vi "WaitOnCommand.vi"(7 "timeout in ms (-1)":i32, 8 "error in (no error)":errorcluster, 10 "queue out":refnum<queue>, 11 "Subsystem in":refnum<class "Subsystem.lvclass">) -> (0 "error out":errorcluster, 2 "element":refnum<class "SubsystemData.lvclass">, 3 "Subsystem out":refnum<class "Subsystem.lvclass">)   [LabVIEW 2017, in "Subsystem.lvclass"]
uses:
  Subsystem.lvclass
  SubsystemData/SubsystemData.lvclass
  Subsystem.lvclass/Subsystem.ctl
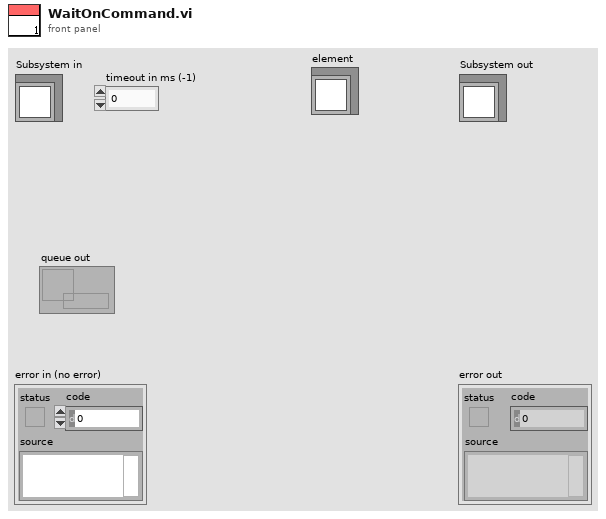
[diagram p1: front panel]
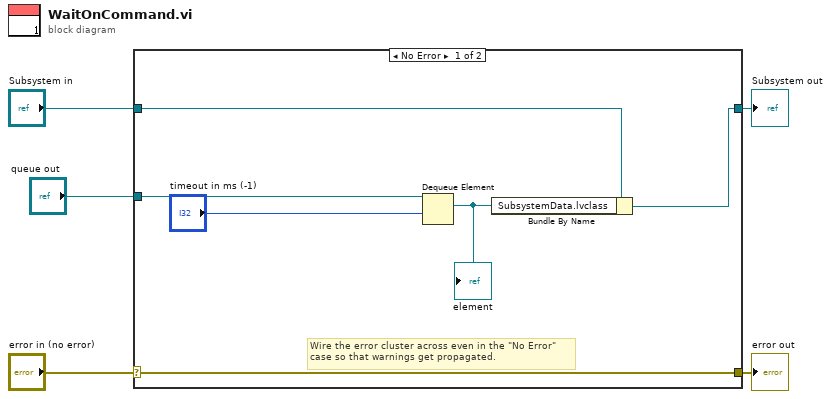
[diagram p0: block diagram]
diagram:
  n1 = case shown="No Error" "error in (no error)" {
    selector: "error in (no error)" -> [w11 w13]
    tunnel: [w11 w13] -> w4
    tunnel: [w6 w12] -> w2
    tunnel: "Subsystem in" -> [w7 w12]
    tunnel: "queue out" -> [w10 _]
    frame No Error {
      # "Wire the error cluster across even in the \"No Error\"\ncase so that warnings get propagated."
      n2 = Dequeue Element(queue=w10, timeout in ms (-1)="timeout in ms (-1)") -> (element=w8:refnum<class "SubsystemData.lvclass">)  [unwired: 1 in, 3 out]
      "element" <- w8
      n3 = Bundle By Name(cluster=w7, "SubsystemData.lvclass"=w8) -> (w6:refnum<class "Subsystem.lvclass">)
    }
    frame Error {
    }
  }
  "error out" <- w4
  "Subsystem out" <- w2
